vi "Read StateManager.vi"(8 "error in (no error)":errorcluster, 11 "Motor in":refnum<class "Motor.lvclass">) -> (0 "error out":errorcluster, 1 "moving":bool, 2 "StateManager":refnum<class "StateManager.lvclass">, 3 "Motor out":refnum<class "Motor.lvclass">, 5 "stateEnum":T1(ring))   [LabVIEW 2018, in "Motor.lvclass"]
uses:
  Motor.lvclass
  StateManager/StateManager.lvclass
  Motor.lvclass/Motor.ctl
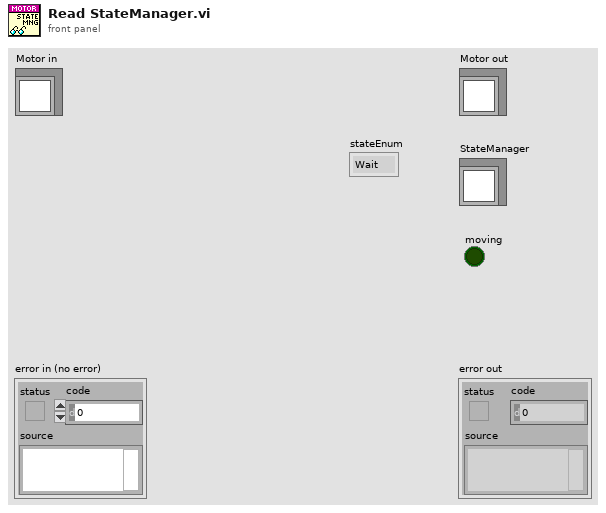
[diagram p1: front panel]
types:
  T1 = enum16{"Wait", "ActiveInit", "ActiveGoto", "ActiveUpdate", "ActiveStop", "ActiveFinish", "SimInit", "SimGoto", "SimUptate", "SimFinish", "CyclicStart", "CyclicUpdate", "CyclicFinish"}
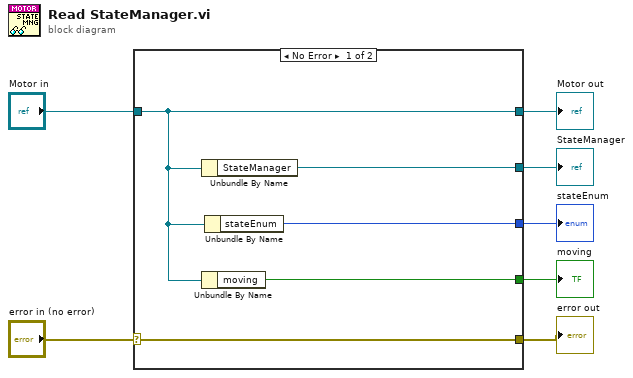
[diagram p0: block diagram]
diagram:
  n1 = case shown="No Error" "error in (no error)" {
    selector: "error in (no error)" -> [w12 w13]
    tunnel: [w12 w13] -> w6
    tunnel: [w9 w14] -> w4
    tunnel: "Motor in" -> [w9 w14]
    tunnel: [w11 _] -> w3
    tunnel: [w10 _] -> w2
    tunnel: [w8 _] -> w1
    frame No Error {
      n2 = Unbundle By Name(w9) -> ("StateManager"=w11:refnum<class "StateManager.lvclass">)
      n3 = Unbundle By Name(w9) -> ("moving"=w10:bool)
      n4 = Unbundle By Name(w9) -> ("stateEnum"=w8:T1)
    }
    frame Error {
    }
  }
  "error out" <- w6
  "Motor out" <- w4
  "StateManager" <- w3
  "moving" <- w2
  "stateEnum" <- w1
